vi "HeaderAction.vi"(0 "InstrClass":refnum<class "Triax320.lvclass"> caption="DNL_LabVIEW Object in", 11 "error in (no error)":errorcluster caption="entrée d'erreur (pas d'erreur)") -> (4 "InstrClassOut":refnum<class "Triax320.lvclass"> caption="DNL_LabVIEW Object out", 6 "DataNames":string[](array[string]), 8 "Instr Name":string, 10 "HeaderString":string, 13 "ArrDisplayNames":string[](array[string]), 14 "DisplayNames":string[](array[string]), 15 "error out":errorcluster caption="sortie d'erreur")   [LabVIEW 2019, in "Triax320.lvclass"]
uses:
  Triax320.lvclass
  C:/Programmes Labview/LabscanV1A/DevicesClass/BaseDevice/BaseDevice.lvclass
  Triax320.lvclass/Triax320.ctl
  <userlib>/Triax320/TriaxParams.ctl
  BaseDevice/BaseDevice.lvclass
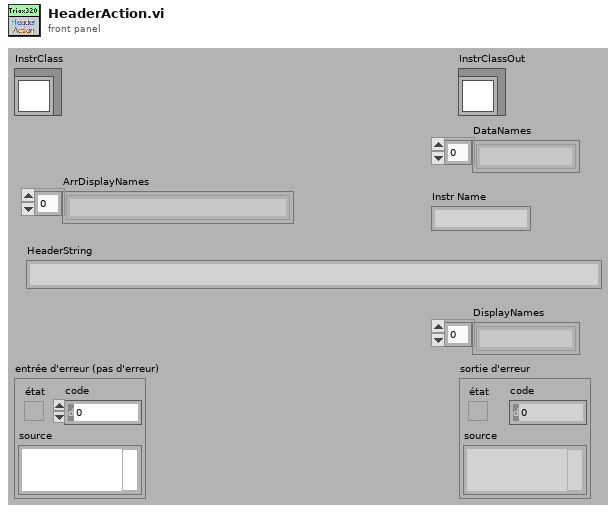
[diagram p1: front panel]
types:
  T1 = typedef "TriaxParams.ctl" = enum16{"Grating", "CalOffset", "Line Density (grv/mm)", "Input Slit (mm)", "Output Slit (mm)", "Both Slit (mm)", "Grating Desc.", "Wavelenght Correction", "Tous"}
  T2 = typedef "Triax320.lvclass/Triax320_Func.ctl" = enum16{"Position (nm)"}
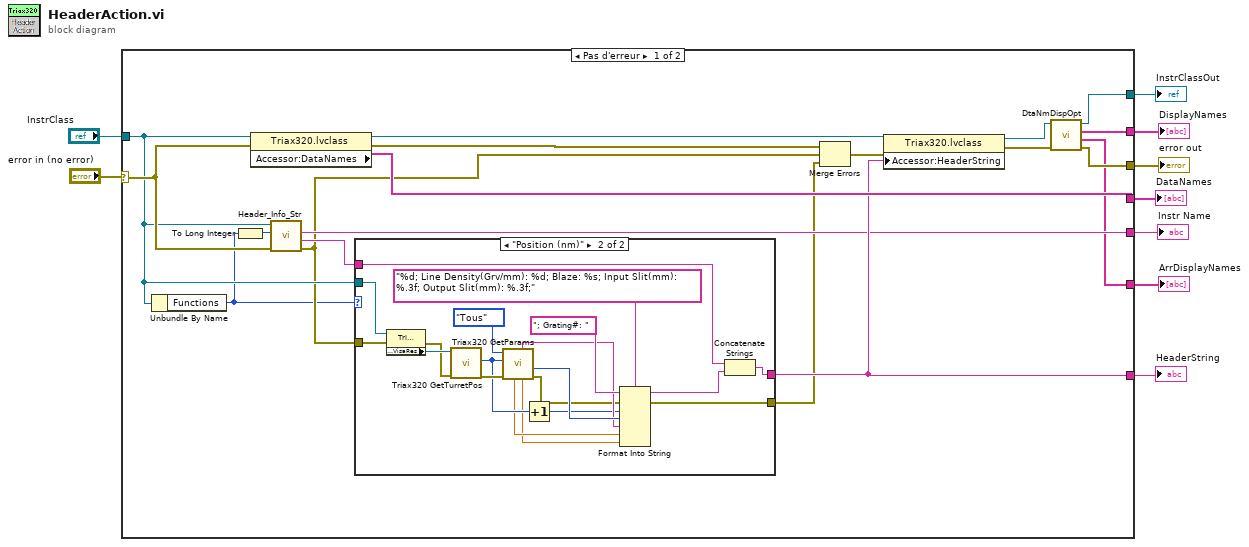
[diagram p0: block diagram]
diagram:
  n1 = case shown="Pas d'erreur" "error in (no error)" {
    selector: "error in (no error)" -> [w17 w50]
    tunnel: [w25 _] -> w8
    tunnel: [w28 _] -> w7
    tunnel: "InstrClass" -> [w15 w51]
    tunnel: [w23 w50] -> w5
    tunnel: [w22 w51] -> w3
    tunnel: [w19 _] -> w4
    tunnel: [w20 _] -> w2
    tunnel: [w10 _] -> w1
    frame No Error {
      n2 = Unbundle By Name(w15) -> ("Functions"=w11:T2)
      n3 = To Long Integer(number=w11) -> (32bit integer=w12:i32)
      n4 = property class="Triax320.lvclass"(reference=w15, error in=w17) -> (reference out=w27:refnum<class "Triax320.lvclass">, error out=w26:errorcluster, "Accessor:DataNames"=w28:string[])
      n5 = call-dynamic "Header_Info_Str.vi"("error in (no error)"=w17, "Functions"=w12, "DefaultDev in"=w15) -> ("error out"=w14:errorcluster, "HdrInfoStr"=w18:string, "InstrumentName"=w19:string)  [unwired: 5 in, 1 out]
      n6 = case shown="\"Position (nm)\"" w11 {
        tunnel: [w30 w47] -> w25
        tunnel: w18 -> [w30 w46]
        tunnel: w15 -> [_ w49]
        tunnel: w14 -> [w29 w48]
        tunnel: [w29 w33] -> w13
        frame Default {
        }
        frame "Position (nm)" {
          n7 = property class="Triax320.lvclass"(reference=w49, error in=w48) -> (error out=w44:errorcluster, "Accessor:VisaRes"=w45:refnum<visa-resource-name>)  [unwired: 1 out]
          n8 = call <userlib>:"Triax320 GetTurretPos.vi"("error in (no error)"=w44, "Triax VISA Rsrc"=w45) -> ("error out"=w43:errorcluster, "Grating"=w41:u8)  [unwired: 7 in, 1 out]
          n9 = call <userlib>:"Triax320 GetParams.vi"("error in"=w43, "Grating"=w41, "Param"=TriaxParams."Tous") -> ("error out"=w34:errorcluster, "LineDensity"=w38:u32, "OutSlit"=w35:dbl, "Grating Description"=w37:string, "InSlit"=w36:dbl)  [unwired: 2 in, 2 out]
          n10 = Increment(x=w41) -> (x+1=w31:u8)
          n11 = Format Into String(format string="%d; Line Density(Grv/mm): %d; Blaze: %s; Input Slit(mm): %.3f; Output Slit(mm): %.3f;" ("chaîne de format"), initial string="; Grating#: " ("chaîne initiale"), error in=w34, w31, w38, w37, w36, w35) -> (resulting string=w32:string, error out=w33:errorcluster)
          n12 = Concatenate Strings(w46, w32) -> (w47:string)
        }
      }
      n13 = Merge Errors(w26, w14, w13) -> (w16:errorcluster)
      n14 = property class="Triax320.lvclass"(reference=w27, error in=w16, "Accessor:HeaderString"=w25) -> (reference out=w21:refnum<class "Triax320.lvclass">, error out=w24:errorcluster)
      n15 = call "DtaNmDispOpt.vi"("error in (no error)"=w24, "BaseDevice en entrée"=w21) -> ("error out"=w23:errorcluster, "ArrDisplayNames"=w10:string[], "DisplayNames"=w20:string[], "BaseDevice en sortie"=w22:refnum<class "Triax320.lvclass">)  [unwired: 6 in]
    }
    frame Error {
    }
  }
  "error out" <- w5
  "InstrClassOut" <- w3
  "DataNames" <- w7
  "HeaderString" <- w8
  "Instr Name" <- w4
  "DisplayNames" <- w2
  "ArrDisplayNames" <- w1
